vi "Avg Loop Rate.vi"(11 "No of Avg":u32=5) -> (3 "Avg Loop Rate":u32)   [LabVIEW 2019]
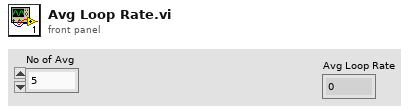
[diagram p1: front panel]
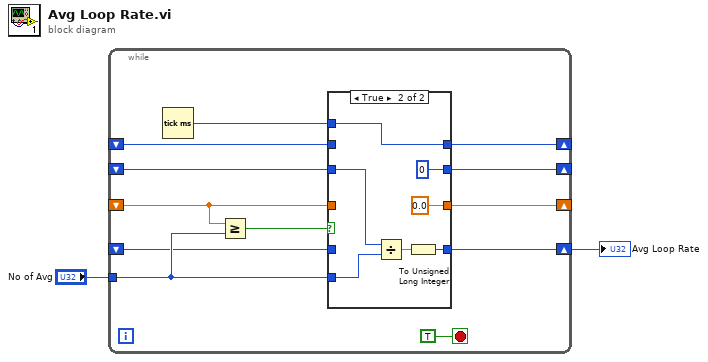
[diagram p0: block diagram]
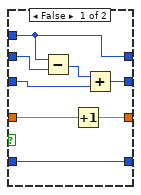
[diagram p2: hidden frame]
diagram:
  n1 = while {
    shift-right: [w5] -> _
    shift-left: _ -> [w4]
    shift-right: [w13] -> _
    shift-left: _ -> [w11]
    tunnel: "No of Avg" -> [w7]
    shift-right: [w9] -> _
    shift-left: _ -> [w8]
    shift-right: [w6] -> w1
    shift-left: _ -> [w3]
    stop <- TRUE stop-if-true
    n2 = Tick Count (ms)() -> (millisecond timer value=w10:u32)
    n3 = Greater Or Equal?(x=w11, y=w7) -> (x >= y?=w12:bool)
    n4 = case shown="True" w12 {
      tunnel: w11 -> [w22 _]
      tunnel: [w21 0.0] -> w13
      tunnel: [w19 w29] -> w5
      tunnel: w10 -> [w19 w29]
      tunnel: w4 -> [w20 _]
      tunnel: [w17 u32 0] -> w9
      tunnel: w8 -> [w16 w26]
      tunnel: w7 -> [_ w25]
      tunnel: [w15 w23] -> w6
      tunnel: w3 -> [w15 _]
      frame False {
        n5 = Subtract(x=w19, y=w20) -> (x-y=w18:u32)
        n6 = Increment(x=w22) -> (x+1=w21:dbl)
        n7 = Add(x=w18, y=w16) -> (x+y=w17:u32)
      }
      frame True {
        n8 = Divide(x=w26, y=w25) -> (x/y=w24:dbl)
        n9 = To Unsigned Long Integer(number=w24) -> (unsigned 32bit integer=w23:u32)
      }
    }
  }
  "Avg Loop Rate" <- w1
